vi "Avantes_SetGet_FGV.vi"(8 "error in":errorcluster, 9 "Set_Get":enum16{"Set", "Get"}(ring)=enum."Get", 11 "in":bool) -> (0 "error out":errorcluster, 3 "out":bool)   [LabVIEW 2011]
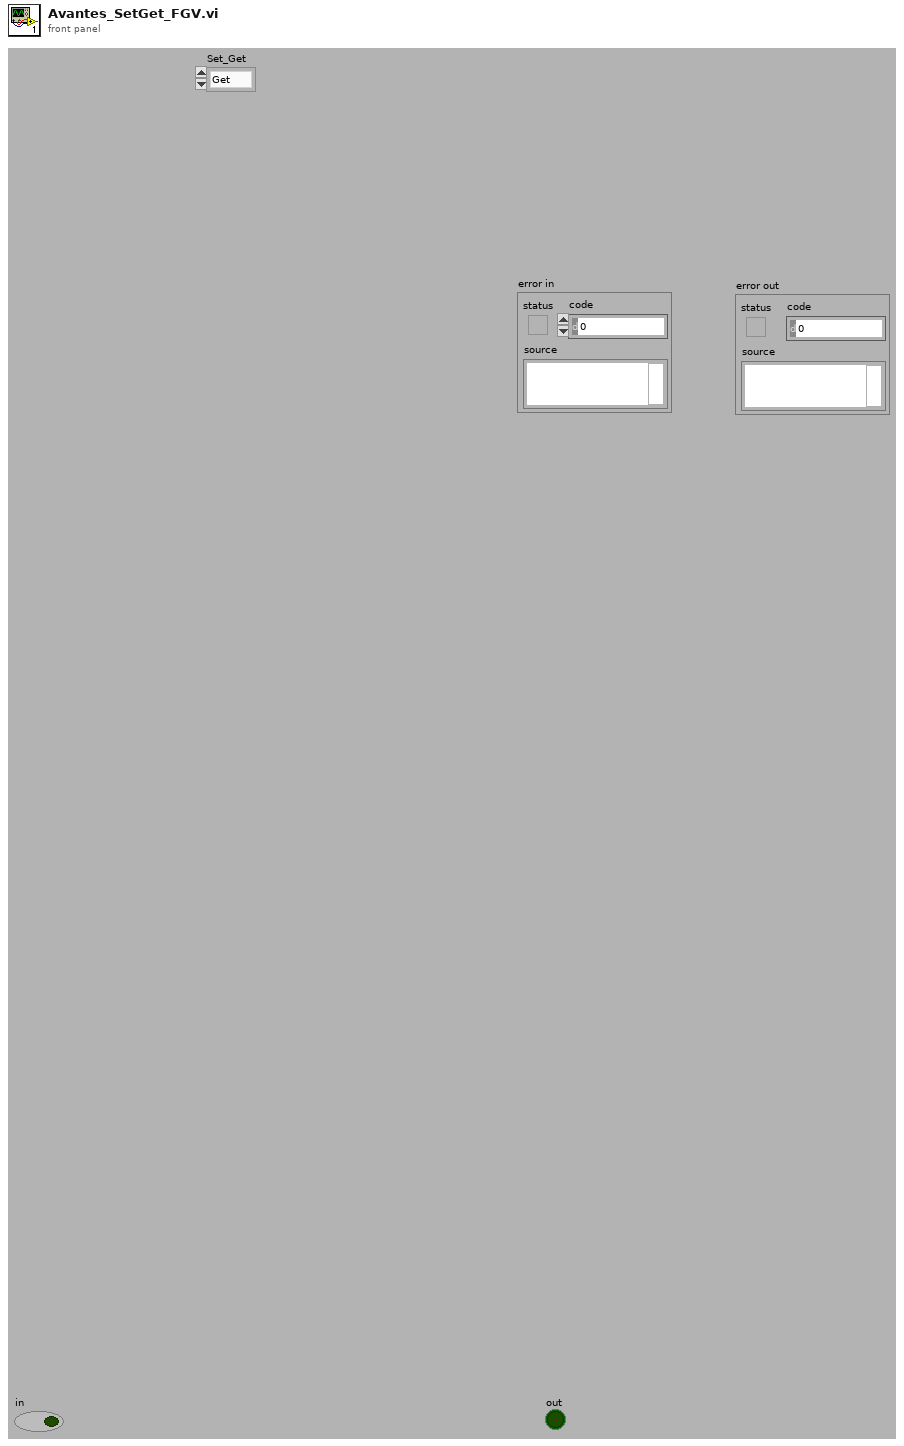
[diagram p1: front panel]
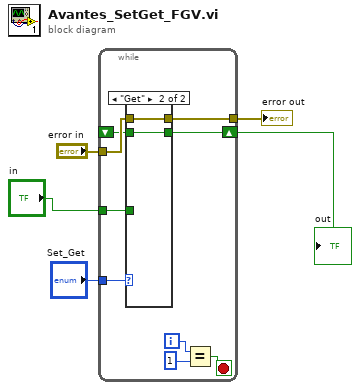
[diagram p0: block diagram]
diagram:
  n1 = while {
    tunnel: "Set_Get" -> [w14]
    tunnel: "error in" -> [w10]
    tunnel: [w9] -> w4
    tunnel: "in" -> [w8]
    shift-right: [w7] -> w1
    shift-left: _ -> [w6]
    i -> [w11]
    stop <- w12 stop-if-true
    n2 = case shown="\"Get\"" w14 {
      tunnel: w10 -> [w16 w18]
      tunnel: [w16 w18] -> w9
      tunnel: w8 -> [w15 _]
      tunnel: [w15 w17] -> w7
      tunnel: w6 -> [_ w17]
      frame "Set", Default {
      }
      frame "Get" {
      }
    }
    n3 = Equal?(x=w11, y=1) -> (x = y?=w12:bool)
  }
  "error out" <- w4
  "out" <- w1
